vi "tm_getdcimgframe.vi"(8 "error in (no error)":errorcluster, 10 "Frame Index":i32=-1, 11 "File Handle in":u32) -> (0 "error out":errorcluster, 1 "Time Sec":dbl, 2 "Data":u16[][](array[numeric]), 3 "File Handle out":u32)   [LabVIEW 2012]
uses:
  tmcamcon.dll
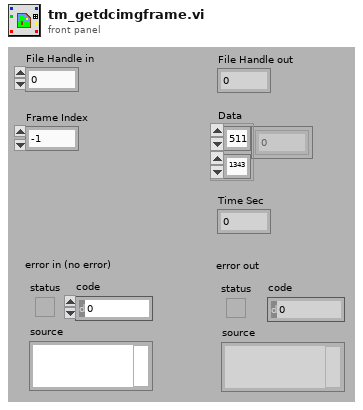
[diagram p1: front panel]
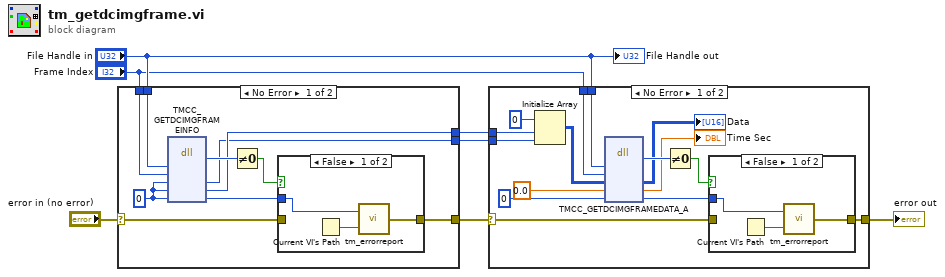
[diagram p0: block diagram]
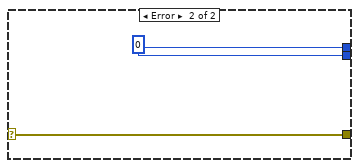
[diagram p5: hidden frame]
diagram:
  n1 = case shown="No Error" "error in (no error)" {
    selector: "error in (no error)" -> [w11 w23]
    tunnel: [w8 w23] -> w6
    tunnel: "File Handle in" -> [w16 _]
    tunnel: [w12 w22] -> w3
    tunnel: [w13 w22] -> w4
    tunnel: "Frame Index" -> [w14 _]
    frame No Error {
      w15 = 0 ("Erval")
      n2 = dll-call lib="tmcamcon.dll" fn="TMCC_GETDCIMGFRAMEINFO"("index"=w16, "frameindex"=w14, "width"=w15, "height"=w15, "Erval"=w15) -> ("return type"=w17:u32, "width"=w12:i32, "height"=w13:i32, "Erval"=w10:i32)  [unwired: 5 in, 2 out]
      n3 = Not Equal To 0?(x=w17) -> (x != 0?=w9:bool)
      n4 = case shown="False" w9 {
        tunnel: w11 -> [_ w21]
        tunnel: [w19 w21] -> w8
        tunnel: w10 -> [w18 _]
        frame False {
          n5 = Current VI's Path() -> (path=w20:path)
          n6 = call "tm_errorreport.vi"("Source"=w20, "Error"=w18) -> ("error out"=w19:errorcluster)
        }
        frame True {
        }
      }
    }
    frame Error {
      w22 = 0 ("buf")
    }
  }
  n7 = case shown="No Error" w6 {
    selector: w6 -> [w27 w43]
    tunnel: [w24 w43] -> w2
    tunnel: "File Handle in" -> [w37 _]
    tunnel: w4 -> [w35 _]
    tunnel: w3 -> [w34 _]
    tunnel: "Frame Index" -> [w31 _]
    frame No Error {
      n8 = Initialize Array(u16 0 ("buf"), w35, w34) -> (w33:u16[][])
      n9 = dll-call lib="tmcamcon.dll" fn="TMCC_GETDCIMGFRAMEDATA_A"("index"=w37, "frame"=w31, "imgarray"=w33, "timestamp"=0.0 ("Erval"), "Erval"=0) -> ("return type"=w38:u32, "imgarray"=→"Data":u16[][], "timestamp"=→"Time Sec":dbl, "Erval"=w26:i32)  [unwired: 5 in, 2 out]
      n10 = Not Equal To 0?(x=w38) -> (x != 0?=w25:bool)
      n11 = case shown="False" w25 {
        tunnel: w27 -> [_ w42]
        tunnel: [w40 w42] -> w24
        tunnel: w26 -> [w39 _]
        frame False {
          n12 = Current VI's Path() -> (path=w41:path)
          n13 = call "tm_errorreport.vi"("Source"=w41, "Error"=w39) -> ("error out"=w40:errorcluster)
        }
        frame True {
        }
      }
    }
    frame Error {
    }
  }
  "error out" <- w2
  "File Handle out" <- "File Handle in"
